vi "Get Service Class Instances.vi"() -> (3 "service instances":refnum<class "ServiceBase.lvclass">[](array[class]))   [LabVIEW 2021, in "ni.measurementlink.measurement.v1.api.lvlib"]
uses:
  ni.measurementlink.measurement.v1.api.lvlib
  <vilib>/gRPC/LabVIEW gRPC Servicer/ServiceBase/ServiceBase.lvclass
  RPC Service/MeasurementService/MeasurementServiceBaseV1.lvclass
  C:/Program Files/National Instruments/LabVIEW 2021/vi.lib/gRPC/LabVIEW gRPC Servicer/ServiceBase/ServiceBase.lvclass
  C:/dev/measurement-plugin-labview/Source/gRPC/Generated APIs/ni/measurementlink/measurement/v1/ni.measurementlink.measurement.v1.api/RPC Service/MeasurementService/MeasurementServiceBaseV1.lvclass
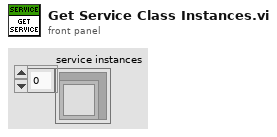
[diagram p1: front panel]
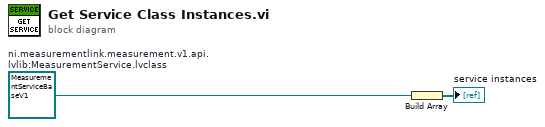
[diagram p0: block diagram]
diagram:
  w1 = refnum<class "MeasurementServiceBaseV1.lvclass"> refnum  # ni.measurementlink.measurement.v1.api.lvlib:MeasurementService.lvclass
  n1 = Build Array(w1) -> (→"service instances":refnum<class "MeasurementServiceBaseV1.lvclass">[])
